vi "16 pulses TX 8spc.vi"(7 "reset system clock":bool, 9 "IQ_run":bool=TRUE, 10 "PDW input Valid":bool, 11 "array PDW":u64[](array[numeric])=[0, 0, 0, 0]) -> (1 "pulse TX status":T1, 2 "output valid":bool, 3 "IQ out":T2[](array[typedef]), 4 "ready for input":bool)   [LabVIEW 2021]
uses:
  <instrlib>/_niInstr/DSP/v1/Shared/Public/IQ Data.ctl
  <instrlib>/_niInstr/Basic Elements/v1/FPGA/Private/Count Up U64.vi
  <instrlib>/_niInstr/Basic Elements/v1/FPGA/Private/Count Up U32.vi
  <instrlib>/_niInstr/Basic Elements/v1/FPGA/niInstr Basic Elements v1 FPGA.lvlib
  <instrlib>/_niInstr/DSP/v1/Shared/niInstr DSP v1 Shared.lvlib
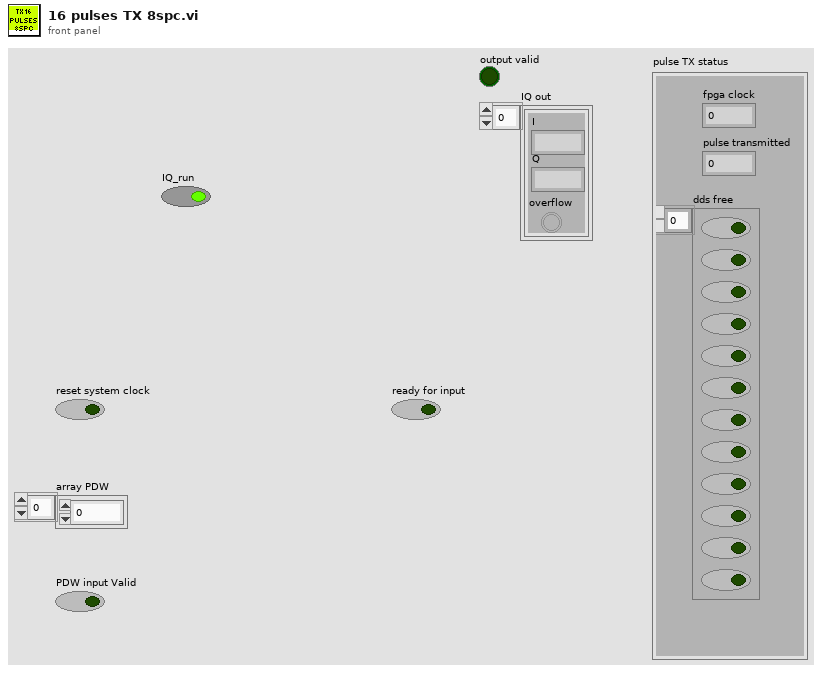
[diagram p1: front panel]
types:
  T1 = cluster{"fpga clock":u64, "pulse transmitted":u32, "dds free":bool[]}
  T2 = typedef "niInstr DSP v1 Shared.lvlib/IQ Data.ctl" = cluster{"I":fxp<+/-,18,1>, "Q":fxp<+/-,18,1>, "overflow":bool}
  T3 = typedef "pdw.ctl" = cluster{"PW":u32, "frequency shift":fxp<+/-,48,0>, "amp":fxp<+/-,18,1>, "mode type":T4, "mode depth":u32, "mode filter":u8, "phase shift":fxp<+/-,16,1>, "pulse shape filter":u8}
  T4 = typedef "mode_type.ctl" = enum8{"CW", "NC - CW", "NC - cw", "LFM", "BPSK", "QPSK"}
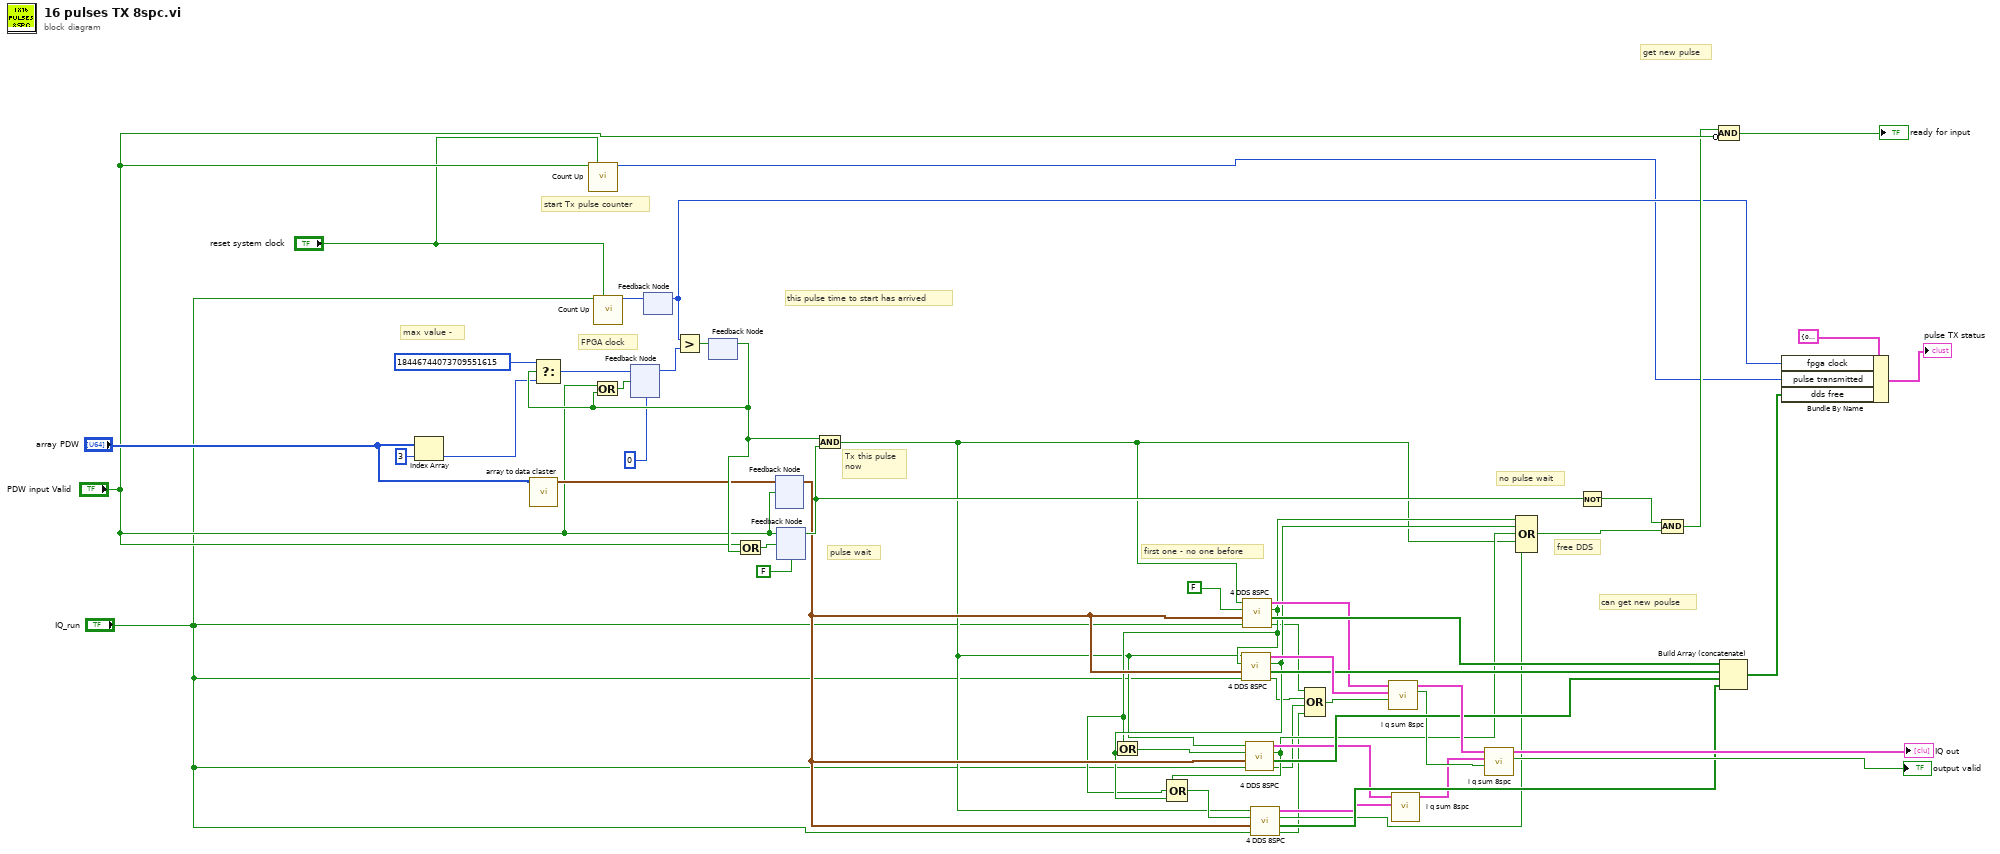
[diagram p0: block diagram]
diagram:
  # "start Tx pulse counter"
  # "FPGA clock"
  # "this pulse time to start has arrived"
  # "first one - no one before"
  # "max value -"
  # "Tx this pulse\nnow"
  # "get new pulse"
  # "pulse wait"
  # "can get new poulse"
  # "no pulse wait"
  # "free DDS"
  n1 = Index Array(array="array PDW", index=3) -> (element=w50:u64)
  n2 = call "array to data claster.vi"("Array"="array PDW") -> ("Cluster"=w43:T3)  [unwired: 10 in]
  n3 = call-poly <instrlib>:"Count Up.vi"("increment"="PDW input Valid", "reset"="reset system clock") -> ("count out"=w3:u32)  [unwired: 13 in]
  n4 = call-poly <instrlib>:"Count Up.vi"("increment"="IQ_run", "reset"="reset system clock") -> ("count out"=w42:u64)  [unwired: 13 in]
  n5 = feedback #1(u64 0 ("U64")) -> (w30:u64)
  n6 = feedback #2() -> (w4:u64)  [unwired: 1 in]
  n7 = feedback-in #2(w42) -> ()
  n8 = Greater?(x=w4, y=w30) -> (0:w53:bool)
  n9 = feedback #3() -> (w54:bool)  [unwired: 1 in]
  n10 = Select(t=u64 18446744073709551615, s=w54, f=w50) -> (s? t:f=w35:u64)
  n11 = Or(x="PDW input Valid", y=w54) -> (x .or. y?=w36:bool)
  n12 = feedback-in #1(w35, w36) -> ()
  n13 = feedback-in #3(w53) -> ()
  n14 = Or(x="PDW input Valid", y=w54) -> (x .or. y?=w40:bool)
  n15 = feedback #4() -> (w18:T3)  [unwired: 1 in]
  n16 = feedback-in #4(w43, "PDW input Valid") -> ()
  n17 = feedback #5(FALSE ("Output Valid")) -> (w47:bool)
  n18 = feedback-in #5("PDW input Valid", w40) -> ()
  n19 = And(x=w54, y=w47) -> (x .and. y?=w12:bool)
  n20 = call "4 DDS 8SPC.vi"("input valid"="IQ_run", "pdw in"=w18, "free DDS before me?"=FALSE, "new PDW in"=w12) -> ("output valid"=w9:bool, "state of every DDS"=w29:bool[], "have free DDS"=w14:bool, "IQ out"=w24:T2[])  [unwired: 4 in]
  n21 = call "4 DDS 8SPC.vi"("input valid"="IQ_run", "pdw in"=w18, "free DDS before me?"=w14, "new PDW in"=w12) -> ("output valid"=w11:bool, "state of every DDS"=w28:bool[], "have free DDS"=w15:bool, "IQ out"=w48:T2[])  [unwired: 4 in]
  n22 = Or(x=w14, y=w15) -> (x .or. y?=w49:bool)
  n23 = call "4 DDS 8SPC.vi"("input valid"="IQ_run", "pdw in"=w18, "free DDS before me?"=w49, "new PDW in"=w12) -> ("output valid"=w8:bool, "state of every DDS"=w27:bool[], "have free DDS"=w13:bool, "IQ out"=w20:T2[])  [unwired: 4 in]
  n24 = Compound Arithmetic op=OR(w13, w14, w15) -> (w16:bool)
  n25 = call "4 DDS 8SPC.vi"("input valid"="IQ_run", "pdw in"=w18, "free DDS before me?"=w16, "new PDW in"=w12) -> ("output valid"=w7:bool, "state of every DDS"=w22:bool[], "have free DDS"=w17:bool, "IQ out"=w21:T2[])  [unwired: 4 in]
  n26 = Compound Arithmetic op=OR(w9, w11, w8, w7) -> (w10:bool)
  n27 = call "i q sum 8spc.vi"("input valid"=w10, "IQ in 2"=w48, "IQ in"=w24) -> ("output valid"=w26:bool, "IQ out"=w45:T2[])  [unwired: 7 in]
  n28 = call "i q sum 8spc.vi"("IQ in 2"=w21, "IQ in"=w20) -> ("IQ out"=w19:T2[])  [unwired: 8 in, 1 out]
  n29 = call "i q sum 8spc.vi"("input valid"=w26, "IQ in 2"=w19, "IQ in"=w45) -> ("output valid"=→"output valid":bool, "IQ out"=→"IQ out":T2[])  [unwired: 7 in]
  n30 = Compound Arithmetic op=OR(w14, w15, w13, w12, w17) -> (w44:bool)
  n31 = Not(x=w47) -> (.not. x?=w31:bool)
  n32 = And(x=w31, y=w44) -> (x .and. y?=w32:bool)
  n33 = Compound Arithmetic op=AND(w32, invert "PDW input Valid") -> (→"ready for input":bool)
  n34 = Build Array (concatenate)(w29, w28, w27, w22) -> (w2:bool[])
  n35 = Bundle By Name(cluster=T1 {"fpga clock"=0, "pulse transmitted"=0, "dds free"=[FALSE, FALSE, FALSE, FALSE, FALSE, FALSE, FALSE, FALSE, FALSE, FALSE, FALSE, FALSE, FALSE, FALSE, FALSE, FALSE]} ("pulse TX status"), "fpga clock"=w4, "pulse transmitted"=w3, "dds free"=w2) -> (→"pulse TX status":T1)
